vi "DataLog Ini.vi"(0 "Auto data log interval":dbl=60.0 min=1.0, 1 "User Data log interval":sgl=5.0 min=0.01 step=0.01, 5 "Datalog directory path":path, 7 "history length":i32=1000 min=1, 9 "graph update interval":dbl=1.0 min=0.0010000000474974513 format="%.2f", 11 "error in (no error)":errorcluster, 12 "Ini Cmd":enum16{"Read", "Write"}(ring)) -> (3 "User Data log interval out":dbl=5.0 min=0.009999999776482582 step=0.009999999776482582, 4 "Auto data log interval out":dbl=60.0 min=1.0, 6 "Datalog directory path out":path, 8 "history length out":i32=1000 min=1, 10 "graph update interval out":dbl=1.0 min=0.0010000000474974513 format="%.2f", 15 "error out":errorcluster)   [LabVIEW 2015]
uses:
  Calibration and Function folders.ctl
  <vilib>/Utility/config.llb/Read Key (Double).vi
  <vilib>/Utility/config.llb/Read Key (Path).vi
  <vilib>/Utility/config.llb/Read Key (I32).vi
  <vilib>/Utility/config.llb/Write Key (Double).vi
  <vilib>/Utility/config.llb/Write Key (Path).vi
  <vilib>/Utility/config.llb/Write Key (I32).vi
  <vilib>/Utility/config.llb/NI_LVConfig.lvlib
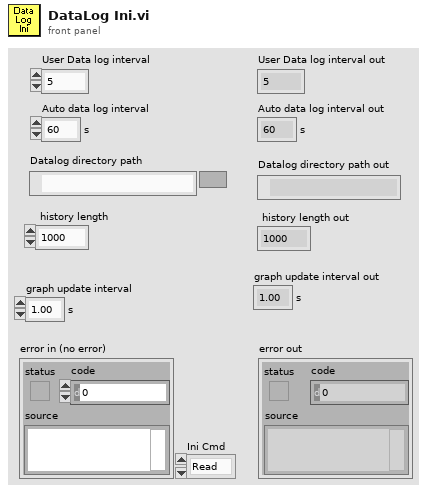
[diagram p1: front panel]
types:
  T1 = typedef "Calibration and Function folders.ctl" = enum16{"Sensors", "Functions", "Config File", "PublicAppFolder", "New ini File", "Set Config File", "Delete ini File"}
  T2 = typedef "NI_LVConfig.lvlib/Config Data RefNum.ctl" = refnum<k1>
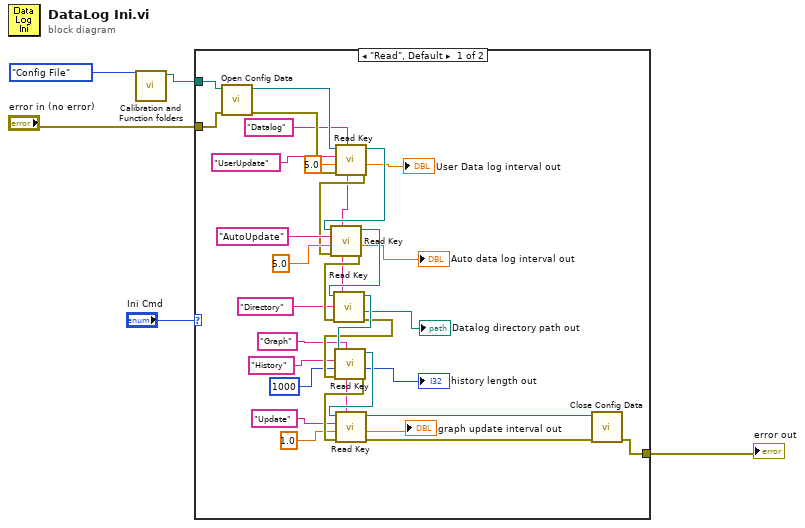
[diagram p0: block diagram]
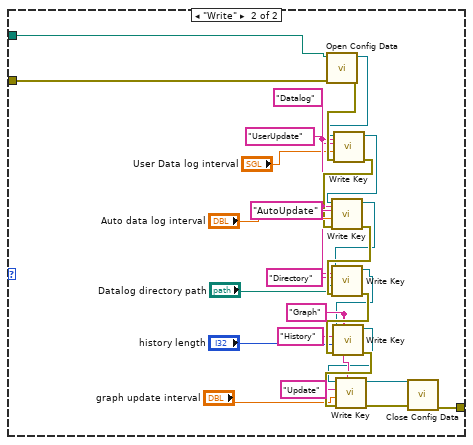
[diagram p2: hidden frame]
diagram:
  n1 = call "Calibration and Function folders.vi"("Folder"=Calibration_and_Function_folders."Config File") -> ("Selected Folder"=w2:path)  [unwired: 9 in, 1 out]
  n2 = case shown="\"Read\", Default" "Ini Cmd" {
    tunnel: "error in (no error)" -> [w35 w46]
    tunnel: [w30 w45] -> w4
    tunnel: w2 -> [w36 w44]
    frame "Read", Default {
      w21 = "Graph" ("section")
      w9 = "Datalog" ("section")
      n3 = call <vilib>:"Open Config Data.vi"("error in (no error)"=w35, "configuration file path"=w36) -> ("error out"=w11:errorcluster, "refnum"=w13:T2)  [unwired: 7 in, 1 out]
      n4 = call-poly <vilib>:"Read Key.vi"("section"=w9, "error in (no error)"=w11, "default value"=5.0, "key"="UserUpdate", "refnum"=w13) -> ("error out"=w10:errorcluster, "value"=→"User Data log interval out":dbl, "refnum out"=w12:T2)  [unwired: 3 in, 1 out]
      n5 = call-poly <vilib>:"Read Key.vi"("section"=w9, "error in (no error)"=w10, "default value"=5.0, "key"="AutoUpdate", "refnum"=w12) -> ("error out"=w28:errorcluster, "value"=→"Auto data log interval out":dbl, "refnum out"=w34:T2)  [unwired: 3 in, 1 out]
      n6 = call-poly <vilib>:"Read Key.vi"("section"=w9, "error in (no error)"=w28, "key"="Directory", "refnum"=w34) -> ("error out"=w27:errorcluster, "value"=→"Datalog directory path out":path, "refnum out"=w33:T2)  [unwired: 4 in, 1 out]
      n7 = call-poly <vilib>:"Read Key.vi"("section"=w21, "error in (no error)"=w27, "default value"=1000, "key"="History", "refnum"=w33) -> ("error out"=w26:errorcluster, "value"=→"history length out":i32, "refnum out"=w32:T2)  [unwired: 3 in, 1 out]
      n8 = call-poly <vilib>:"Read Key.vi"("section"=w21, "error in (no error)"=w26, "default value"=1.0, "key"="Update", "refnum"=w32) -> ("error out"=w29:errorcluster, "value"=→"graph update interval out":dbl, "refnum out"=w31:T2)  [unwired: 3 in, 1 out]
      n9 = call <vilib>:"Close Config Data.vi"("error in (no error)"=w29, "refnum"=w31) -> ("error out"=w30:errorcluster)  [unwired: 8 in, 1 out]
    }
    frame "Write" {
      w59 = "Graph" ("section")
      w39 = "Datalog" ("section")
      n10 = call <vilib>:"Open Config Data.vi"("error in (no error)"=w46, "configuration file path"=w44) -> ("error out"=w43:errorcluster, "refnum"=w41:T2)  [unwired: 7 in, 1 out]
      n11 = call-poly <vilib>:"Write Key.vi"("section"=w39, "error in (no error)"=w43, "value"="User Data log interval", "key"="UserUpdate", "refnum"=w41) -> ("error out"=w42:errorcluster, "refnum out"=w40:T2)  [unwired: 4 in, 1 out]
      n12 = call-poly <vilib>:"Write Key.vi"("section"=w39, "error in (no error)"=w42, "value"="Auto data log interval", "key"="AutoUpdate", "refnum"=w40) -> ("error out"=w62:errorcluster, "refnum out"=w58:T2)  [unwired: 4 in, 1 out]
      n13 = call-poly <vilib>:"Write Key.vi"("section"=w39, "error in (no error)"=w62, "value"="Datalog directory path", "key"="Directory", "refnum"=w58) -> ("error out"=w61:errorcluster, "refnum out"=w57:T2)  [unwired: 4 in, 1 out]
      n14 = call-poly <vilib>:"Write Key.vi"("section"=w59, "error in (no error)"=w61, "value"="history length", "key"="History", "refnum"=w57) -> ("error out"=w60:errorcluster, "refnum out"=w56:T2)  [unwired: 4 in, 1 out]
      n15 = call-poly <vilib>:"Write Key.vi"("section"=w59, "error in (no error)"=w60, "value"="graph update interval", "key"="Update", "refnum"=w56) -> ("error out"=w55:errorcluster, "refnum out"=w54:T2)  [unwired: 4 in, 1 out]
      n16 = call <vilib>:"Close Config Data.vi"("error in (no error)"=w55, "refnum"=w54) -> ("error out"=w45:errorcluster)  [unwired: 8 in, 1 out]
    }
  }
  "error out" <- w4
